vi "【仿真】1个数据采集模块8个被击打部位n次击打.vi"() -> ()   [LabVIEW 2010]
uses:
  <vilib>/Waveform/WDTFileIO.llb/Export Waveform To Spreadsheet File.vi
  <vilib>/Analysis/NI_AALBase.lvlib
panel:
  in  "选项卡控件":enum32{"初始设置及运行中数据", "统计结果"}(tab)
  in  "设置传感器瞬时记录及测试报告存储路径":path
  out "第几次击打":i32
  out "传感器实时力值":dbl(graph)
  out "本次击打反应时间":dbl
  in  "设置击打次数":u8=1 min=1 step=1
  in  "设置两次击打间隔时间（秒）":sgl min=0.1
  out "击打部位编号":dbl
  out "本次击打最大力值":dbl caption="本次击打力值" format="%0.2f"
  out "平均值":dbl caption="均值" format="%0.2f"
  out "最大值":dbl
  out "最小值":dbl
  out "最慢":dbl
  out "最快":dbl
  out "反应时间平均值":dbl caption="平均" format="%0.2f"
  out "力值直方图":T1(graph) caption="力直方图"
  # "第"
  # "次击打"
  # "力"
  # "反应时间"
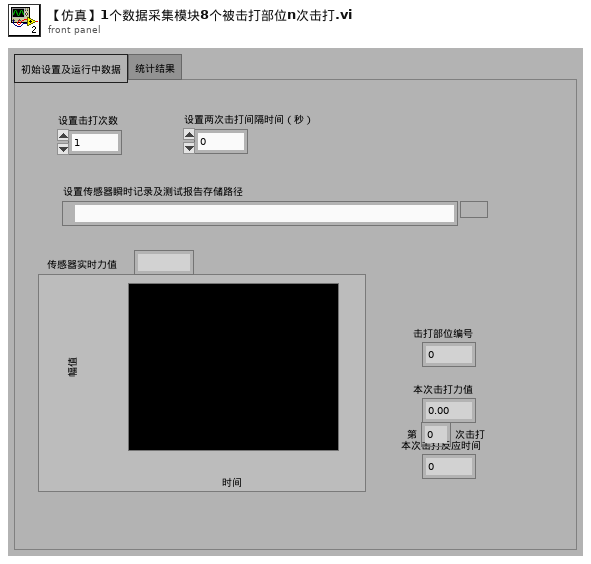
[diagram p1: front panel]
types:
  T1 = cluster{"X Values":dbl[], "Histogram: h(x)":i32[]}
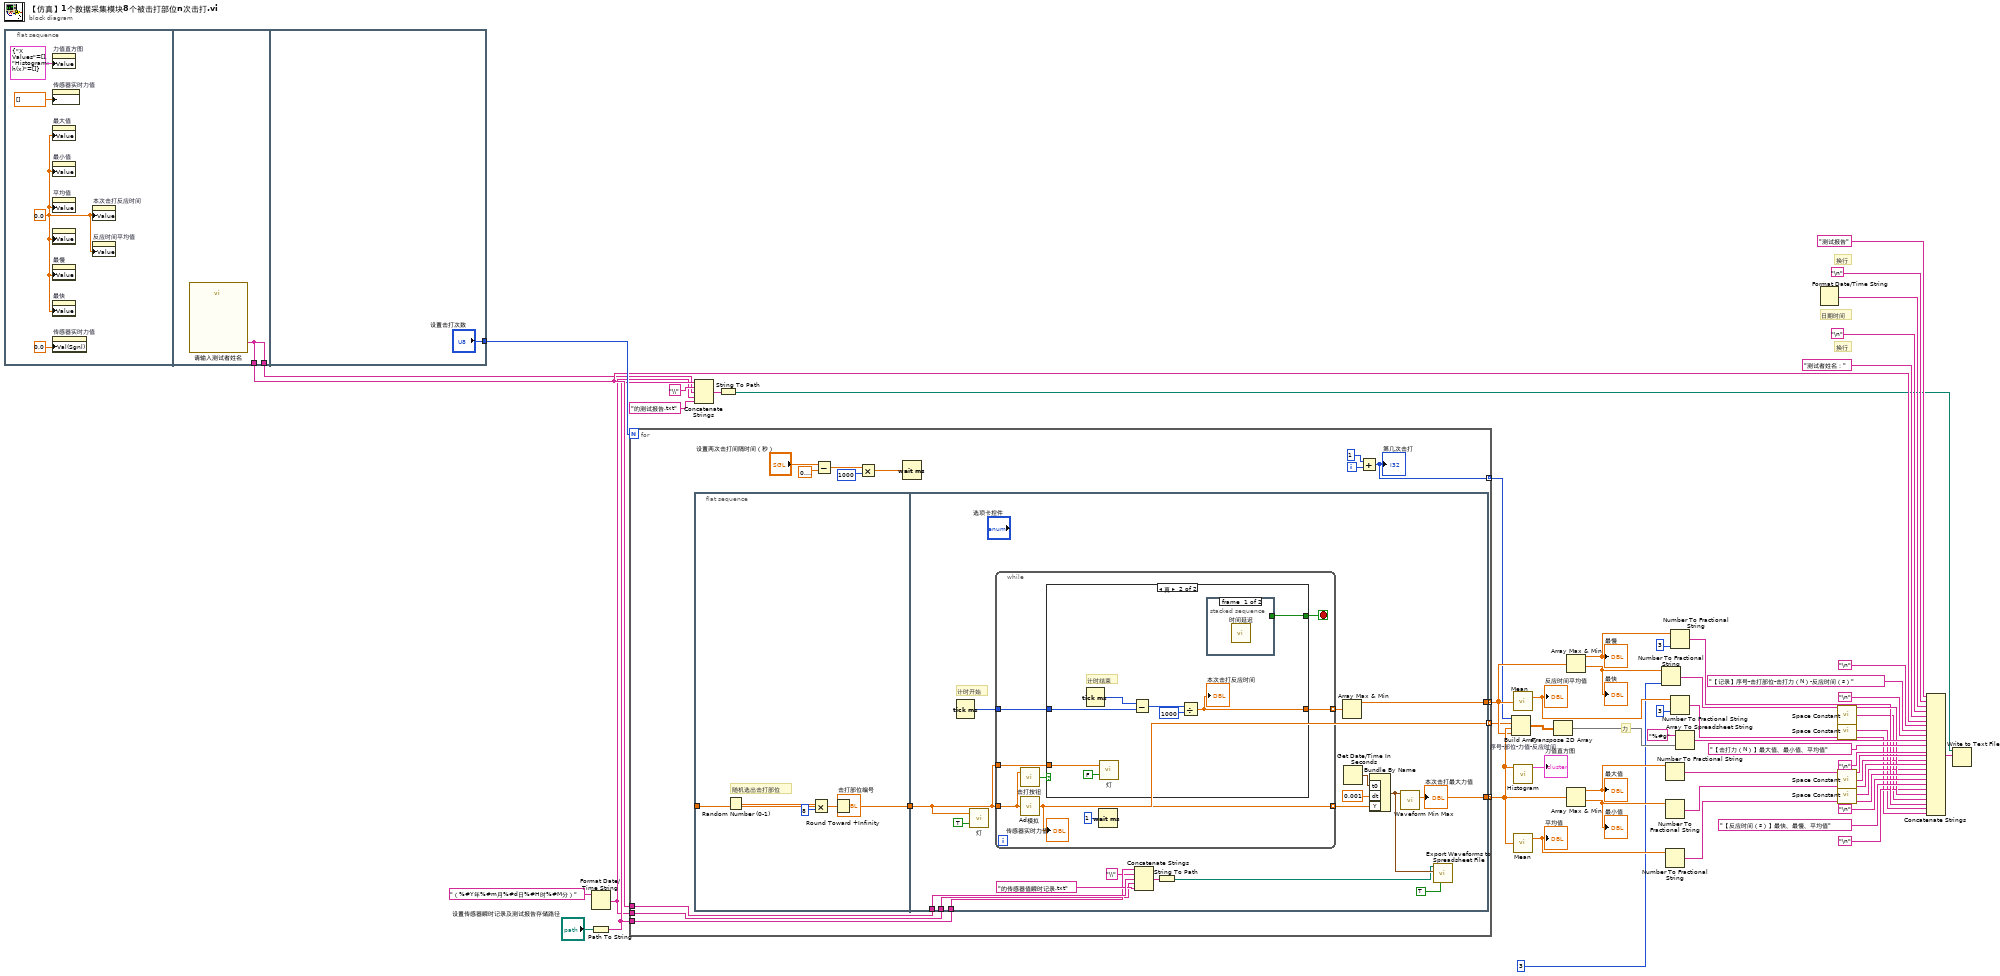
[diagram p0: block diagram]
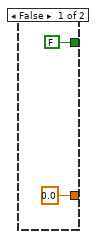
[diagram p2: hidden frame]
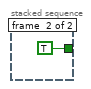
[diagram p3: hidden frame]
diagram:
  # "换行"
  # "日期时间"
  # "换行"
  # "力"
  n1 = flat-sequence {
    tunnel: [w58] -> w26
    tunnel: [w58] -> w4
    tunnel: ["设置击打次数"] -> w27
    frame #0 {
      w54 = 0.0 ("实时力值")
      n2 = property on="力值直方图" class="XYGraph (严格)"("Value"=T1 {"X Values"=[], "Histogram: h(x)"=[]} ("力值直方图")) -> ()  [unwired: 2 in, 2 out]
      n3 = property on="传感器实时力值" class="WFChart (严格)"("History Data"=dbl[] [] ("历史数据")) -> ()  [unwired: 2 in, 2 out]
      n4 = property on="最大值" class="DigNum (严格)"("Value"=w54) -> ()  [unwired: 2 in, 2 out]
      n5 = property on="最小值" class="DigNum (严格)"("Value"=w54) -> ()  [unwired: 2 in, 2 out]
      n6 = property on="平均值" class="DigNum (严格)"("Value"=w54) -> ()  [unwired: 2 in, 2 out]
      n7 = property class="DigNum (严格)"("Value"=w54) -> ()  [unwired: 2 in, 2 out]
      n8 = property on="最慢" class="DigNum (严格)"("Value"=w54) -> ()  [unwired: 2 in, 2 out]
      n9 = property on="最快" class="DigNum (严格)"("Value"=w54) -> ()  [unwired: 2 in, 2 out]
      n10 = property on="传感器实时力值" class="WFChart (严格)"("Val(Sgnl)"=0.0 ("值(信号)")) -> ()  [unwired: 2 in, 2 out]
      n11 = property on="本次击打反应时间" class="DigNum (严格)"("Value"=w54) -> ()  [unwired: 2 in, 2 out]
      n12 = property on="反应时间平均值" class="DigNum (严格)"("Value"=w54) -> ()  [unwired: 2 in, 2 out]
    }
    frame #1 {
      n13 = call "请输入测试者姓名"() -> ("姓名"=w58:string)  [unwired: 17 in, 2 out]
    }
    frame #2 {
    }
  }
  n14 = Format Date/Time String(time format string (%c)="（%#Y年%#m月%#d日%#H时%#M分）" ("时间格式字符串(%c)")) -> (date/time string=w3:string)  [unwired: 2 in]
  n15 = Path To String(path="设置传感器瞬时记录及测试报告存储路径") -> (string=w9:string)
  n16 = for {
    N: w27 -> [_]
    tunnel: [w71] -> w6 mode=indexing
    tunnel: [w70] -> w5 mode=indexing
    tunnel: w26 -> [w69]
    tunnel: w9 -> [w63]
    tunnel: w3 -> [w62]
    tunnel: [w61] -> w2 mode=indexing
    tunnel: [w60] -> w1 mode=indexing
    i -> [w65]
    n17 = flat-sequence {
      tunnel: [w75] -> w74
      tunnel: [w75] -> w60
      tunnel: w74 -> [w89]
      tunnel: [w91] -> w71
      tunnel: [w87] -> w70
      tunnel: w69 -> [w85]
      tunnel: w63 -> [w81]
      tunnel: w62 -> [w79]
      frame #0 {
        # "随机选出击打部位"
        n18 = Random Number (0-1)() -> (number: 0 to 1=w78:dbl)
        n19 = Multiply(x=w78, y=u8 8) -> (x*y=w76:dbl)
        n20 = Round Toward +Infinity(x=w76) -> (ceil(x): smallest int >= x=w75:dbl)
        "击打部位编号" <- w75
      }
      frame #1 {
        # "计时开始"
        n21 = Tick Count (ms)() -> (millisecond timer value=w90:u32)
        n22 = call "灯.vi"("输入值T/F"=TRUE ("开关量值"), "Set_Do_通道号（灯号）"=w89) -> ()  [unwired: 1 in]
        n23 = while {
          tunnel: w89 -> [w97]
          tunnel: [w103] -> w94 mode=indexing
          tunnel: w90 -> [w101]
          tunnel: w89 -> [w102]
          tunnel: [w99] -> w88 mode=indexing
          stop <- w100 stop-if-true
          n24 = call "击打按钮.vi"("Get_Di_通道号"=w97) -> ("返回值（点亮为返回T）"=w98:bool)  [unwired: 1 in]
          n25 = call "Ad模拟.vi"("Ad通道号"=w97) -> ("仿真值"=w103:dbl)
          "传感器实时力值" <- w103
          n26 = case shown="真" w98 {
            tunnel: w102 -> [_ w110]
            tunnel: w101 -> [_ w109]
            tunnel: [FALSE w108] -> w100
            tunnel: [0.0 w107] -> w99
            frame False {
            }
            frame True {
              # "计时结束"
              n27 = Tick Count (ms)() -> (millisecond timer value=w111:u32)
              n28 = call "灯.vi"("输入值T/F"=FALSE, "Set_Do_通道号（灯号）"=w110) -> ()  [unwired: 1 in]
              n29 = Subtract(x=w111, y=w109) -> (x-y=w112:u32)
              n30 = Divide(x=w112, y=u32 1000) -> (x/y=w107:dbl)
              "本次击打反应时间" <- w107
              n31 = stacked-sequence {
                tunnel: [_ TRUE] -> w108
                frame #0 {
                  n32 = call "时间延迟"() -> ()  [unwired: 11 in, 1 out]
                }
                frame #1 {
                }
              }
            }
          }
          n33 = Wait (ms)(milliseconds to wait=u32 1 ("等待时间（毫秒）")) -> ()  [unwired: 1 out]
        }
        n34 = Concatenate Strings(w81, "\\" ("字符串"), w85, w79, "的传感器值瞬时记录.txt" ("字符串")) -> (w84:string)
        n35 = String To Path(string=w84) -> (path=w83:path)
        n36 = Array Max & Min(array=w88) -> (max value=w87:dbl)  [unwired: 3 out]
        n37 = Get Date/Time In Seconds() -> (seconds since 1Jan1904=w86:timestamp)
        n38 = Bundle By Name("t0"=w86, "dt"=0.001, "Y"=w94) -> (w92:waveform(dbl))  [unwired: 1 in]
        n39 = call <vilib>:"Waveform Min Max.vi"("waveform in"=w92) -> ("Y max"=w91:dbl)  [unwired: 5 in, 5 out]
        "本次击打最大力值" <- w91
        n40 = call-poly <vilib>:"Export Waveforms to Spreadsheet File.vi"("append to file? (new file:F)"=TRUE, "waveform"=w92, "file path (dialog if empty)"=w83) -> ()  [unwired: 7 in, 2 out]
      }
    }
    n41 = Subtract(x="设置两次击打间隔时间（秒）", y=sgl 0.1) -> (x-y=w66:sgl)
    n42 = Multiply(x=w66, y=u32 1000) -> (x*y=w73:sgl)
    n43 = Wait (ms)(milliseconds to wait=w73) -> ()  [unwired: 1 out]
    n44 = Add(x=1, y=w65) -> (x+y=w61:i32)
    "第几次击打" <- w61
  }
  n45 = Concatenate Strings(w9, "\\" ("字符串"), w4, w3, "的测试报告.txt" ("字符串")) -> (w10:string)
  n46 = String To Path(string=w10) -> (path=w7:path)
  n47 = Build Array "序号-部位-力值-反应时间"(w2, w1, w6, w5) -> (w20:dbl[][])
  n48 = call <vilib>:"Mean.vi"("X"=w5) -> ("mean"=w17:dbl)  [unwired: 1 out]
  "反应时间平均值" <- w17
  n49 = call <vilib>:"Mean.vi"("X"=w6) -> ("mean"=w48:dbl)  [unwired: 1 out]
  "平均值" <- w48
  n50 = call <vilib>:"Histogram.vi"("X"=w6) -> ("Histogram Graph"=→"力值直方图":T1)  [unwired: 7 in, 3 out]
  n51 = Transpose 2D Array(2D array=w20) -> (transposed array=w19:dbl[][])
  n52 = Array Max & Min(array=w5) -> (max value=w46:dbl, min value=w47:dbl)  [unwired: 2 out]
  "最慢" <- w46
  "最快" <- w47
  n53 = Array Max & Min(array=w6) -> (max value=w50:dbl, min value=w49:dbl)  [unwired: 2 out]
  "最大值" <- w50
  "最小值" <- w49
  n54 = Number To Fractional String(number=w47, precision (6)=i16 3 ("精度(6)")) -> (F-format string=w29:string)  [unwired: 2 in]
  n55 = Number To Fractional String(number=w50) -> (F-format string=w34:string)  [unwired: 3 in]
  n56 = Number To Fractional String(number=w49) -> (F-format string=w33:string)  [unwired: 3 in]
  n57 = Number To Fractional String(number=w48) -> (F-format string=w32:string)  [unwired: 3 in]
  n58 = Number To Fractional String(number=w46, precision (6)=i16 3 ("精度(6)")) -> (F-format string=w28:string)  [unwired: 2 in]
  n59 = Number To Fractional String(number=w17, precision (6)=i16 3 ("精度(6)")) -> (F-format string=w18:string)  [unwired: 2 in]
  n60 = Array To Spreadsheet String(array=w19, 3:"%#g" ("格式字符串")) -> (spreadsheet string=w37:string)  [unwired: 1 in]
  n61 = Format Date/Time String() -> (date/time string=w43:string)  [unwired: 3 in]
  n62 = call <vilib>:"Space Constant.vi"() -> ("String"=w21:string)
  n63 = call <vilib>:"Space Constant.vi"() -> ("String"=w22:string)
  n64 = call <vilib>:"Space Constant.vi"() -> ("String"=w24:string)
  n65 = call <vilib>:"Space Constant.vi"() -> ("String"=w23:string)
  n66 = Concatenate Strings("测试报告", "\n", w43, "\n", "测试者姓名：", w26, "\n", "【记录】序号-击打部位-击打力（N）-反应时间（s）", "\n", w37, "【击打力（N）】最大值、最小值、平均值", "\n", w34, w24, w33, w23, w32, "\n", "【反应时间（s）】最快、最慢、平均值", "\n", w29, w21, w28, w22, w18) -> (w52:string)
  n67 = Write to Text File(file (use dialog)=w7, text=w52) -> ()  [unwired: 2 in, 3 out]
